vi "PeriodicUpdates.vi"(8 "error in (no error)":errorcluster, 11 "Gserver in":refnum<class "Gserver.lvclass">) -> (0 "error out":errorcluster, 3 "Gserver out":refnum<class "Gserver.lvclass">)   [LabVIEW 2020, in "Gserver.lvclass"]
doc: "Andre Koelewijn, 18 jan 2021\n\nSent out periodic Gviewer updates for Live mode"
uses:
  Gserver.lvclass
  Gserver.lvclass/Gserver.ctl
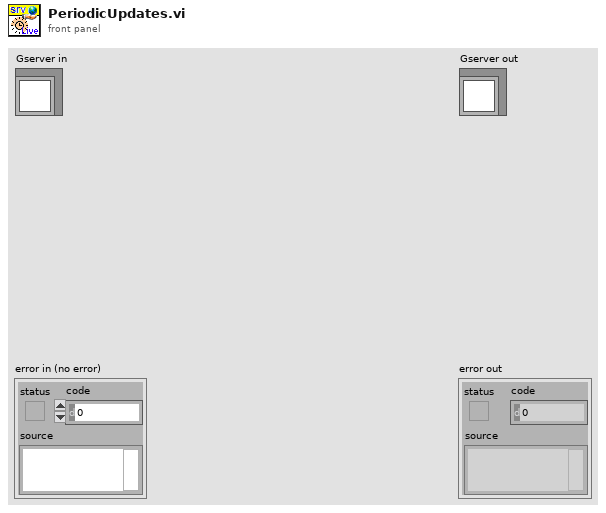
[diagram p1: front panel]
types:
  T1 = typedef "Gserver.lvclass/Typedef_PeriodicUpdate.ctl" = cluster{"Sending Gviewer":string, "PreviousUpdate":timestamp, "UpdateRate":dbl, "DataRequest":T2}
  T2 = typedef "Gviewer.lvclass/Typedef_datarequest.ctl" = cluster{"Tags":string[], "Live":T3, "Time-Start":timestamp, "Time-End":timestamp, "TimeSpan":dbl, "DisplayResolution":i32}
  T3 = typedef "Gviewer.lvclass/Typedef_Live.ctl" = enum16{"Live View", "Freeze"}
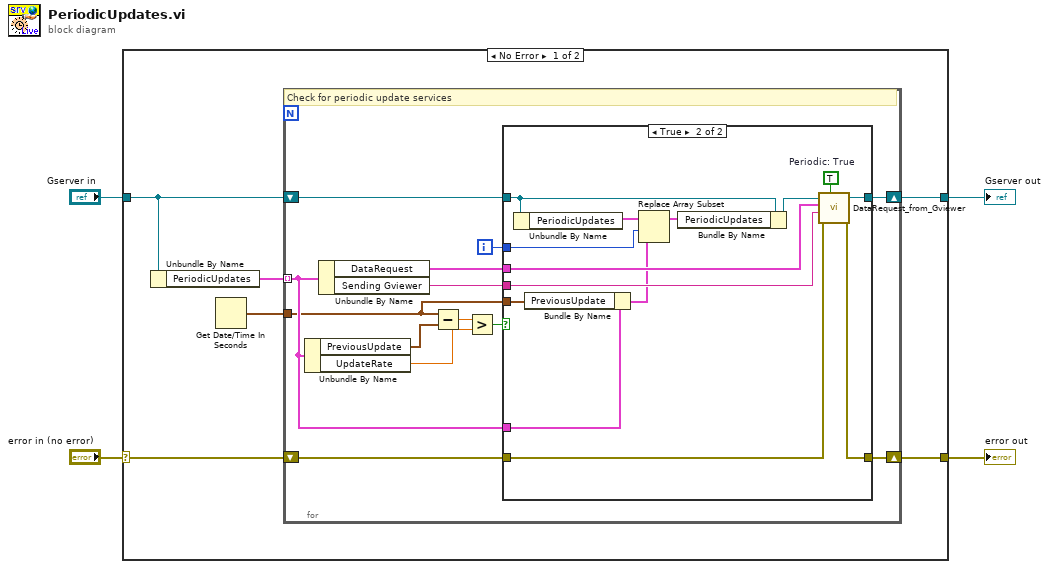
[diagram p0: block diagram]
diagram:
  n1 = case shown="No Error" "error in (no error)" {
    selector: "error in (no error)" -> [w6 w41]
    tunnel: [w5 w41] -> w3
    tunnel: [w8 w40] -> w1
    tunnel: "Gserver in" -> [w7 w40]
    frame No Error {
      n2 = Unbundle By Name(w7) -> ("PeriodicUpdates"=w10:T1[])
      n3 = Get Date/Time In Seconds() -> (seconds since 1Jan1904=w9:timestamp)
      n4 = for {
        tunnel: w10 -> [w13] mode=indexing
        tunnel: w9 -> [w12]
        shift-right: [w18] -> w8
        shift-left: w7 -> [w19]
        shift-right: [w16] -> w5
        shift-left: w6 -> [w17]
        i -> [w11]
        # "Check for periodic update services"
        n5 = Unbundle By Name(w13) -> ("PreviousUpdate"=w23:timestamp, "UpdateRate"=w21:dbl)
        n6 = Unbundle By Name(w13) -> ("DataRequest"=w14:T2, "Sending Gviewer"=w15:string)
        n7 = Subtract(x=w12, y=w23) -> (x-y=w22:dbl)
        n8 = Greater?(x=w22, y=w21) -> (0:w20:bool)
        n9 = case shown="True" w20 {
          tunnel: w19 -> [w25 w26]
          tunnel: [w25 w32] -> w18
          tunnel: w17 -> [w24 w39]
          tunnel: [w24 w38] -> w16
          tunnel: w15 -> [_ w37]
          tunnel: w14 -> [_ w36]
          tunnel: w13 -> [_ w34]
          tunnel: w12 -> [_ w33]
          tunnel: w11 -> [_ w30]
          frame False {
          }
          frame True {
            w35 = TRUE  # Periodic: True
            n10 = Unbundle By Name(w26) -> ("PeriodicUpdates"=w31:T1[])
            n11 = Bundle By Name(cluster=w34, "PreviousUpdate"=w33) -> (w29:T1)
            n12 = Replace Array Subset(array=w31, new element=w29, index=w30) -> (w28:T1[])
            n13 = Bundle By Name(cluster=w26, "PeriodicUpdates"=w28) -> (w27:refnum<class "Gserver.lvclass">)
            n14 = call "DataRequest_from_Gviewer.vi"("Periodic?"=w35, "error in (no error)"=w39, "Sending Gviewer"=w37, "DataRequest"=w36, "Gserver in"=w27) -> ("error out"=w38:errorcluster, "Gserver out"=w32:refnum<class "Gserver.lvclass">)  [unwired: 5 in]
          }
        }
      }
    }
    frame Error {
    }
  }
  "error out" <- w3
  "Gserver out" <- w1
